vi "AB_Log_Linker_Item.vi"(6 "inclusion":T1, 7 "comment":string, 8 "error in (no error)":errorcluster, 9 "index":i32, 10 "linkerItem":T3, 11 "AB_Source.lvclass":refnum<class "AB_Source.lvclass">) -> (0 "error out":errorcluster)   [LabVIEW 2020]
uses:
  <vilib>/AppBuilder/AB_Classes/Source/AB_Source.lvclass
  <vilib>/Utility/lvfile.llb/LVFileType.ctl
  <vilib>/AppBuilder/Engine/AB_Engine_Linker_Inclusion.ctl
  <vilib>/Utility/lvfile.llb/NI_FileType.lvlib
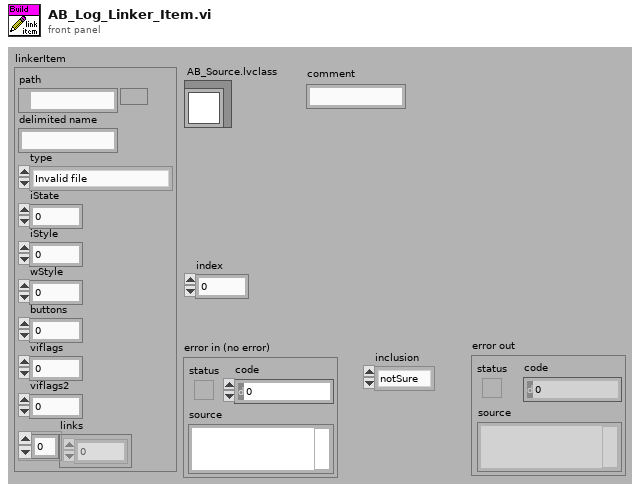
[diagram p1: front panel]
types:
  T1 = typedef "AB_Engine_Linker_Inclusion.ctl" = enum16{"notSure", "include", "exclude", "excludeChild"}
  T2 = typedef "NI_FileType.lvlib/LVFileType.ctl" = enum32{"Invalid file", "Unknown type", "Instrument", "Control", "Polymorphic VI", "Project", "Library", "LVClass", "XControl", "XNode", "Shared library", ".NET assembly", "ActiveX interface", "CIN", "Run-time menu", "Palette menu", "Help file", "LLB", "XNode Edit Dependency", "Class Private Data Control", "Statechart", "MathScript .m file", "Ladder Diagram", "LVLibp", "XNode Build Dependency"}
  T3 = cluster{"path":path, "delimited name":string, "type":T2, "iState":u32, "iStyle":u16, "wStyle":u16, "buttons":u16, "viflags":u32, "viflags2":u32, "links":u32[]}
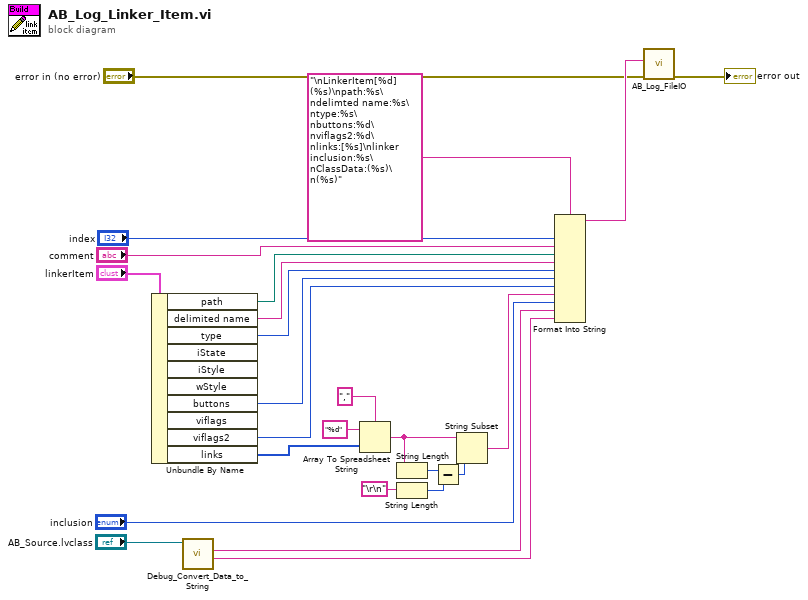
[diagram p0: block diagram]
diagram:
  n1 = Unbundle By Name("linkerItem") -> ("path"=w16:path, "delimited name"=w15:string, "type"=w14:T2, "buttons"=w13:u16, "viflags2"=w12:u32, "links"=w17:u32[])  [unwired: 4 out]
  n2 = call-dynamic "Debug_Convert_Data_to_String.vi"("AB_Source in"="AB_Source.lvclass") -> ("classData"=w1:string, "sourceType"=w9:string)  [unwired: 7 in, 2 out]
  n3 = Array To Spreadsheet String(delimiter (Tab)=",", array=w17, 3:"%d" ("format string")) -> (spreadsheet string=w3:string)
  n4 = String Length(string=w3) -> (length=w6:i32)
  n5 = String Length(string="\r\n") -> (length=w5:i32)
  n6 = Subtract(x=w6, y=w5) -> (x-y=w4:i32)
  n7 = String Subset(string=w3, length (rest)=w4) -> (substring=w2:string)  [unwired: 1 in]
  n8 = Format Into String(format string="\nLinkerItem[%d] (%s)\npath:%s\ndelimted name:%s\ntype:%s\nbuttons:%d\nviflags2:%d\nlinks:[%s]\nlinker inclusion:%s\nClassData:(%s)\n(%s)", "index", "comment", w16, w15, w14, w13, w12, w2, "inclusion", w9, w1) -> (resulting string=w24:string)  [unwired: 2 in, 1 out]
  n9 = call <vilib>:"AB_Log_FileIO.vi"("error in (no error)"="error in (no error)", "data"=w24) -> ("error out"=→"error out":errorcluster)  [unwired: 9 in]
